vi "get property.vi"(0 "reference in":refnum<class "TDMS_DataHandler.lvclass">, 2 "Combo Box":T1, 5 "error in (no error)":errorcluster) -> (14 "reference out":refnum<class "TDMS_DataHandler.lvclass">, 16 "data":string, 19 "error out":errorcluster)   [LabVIEW 2019, in "TDMS_DataHandler.lvclass"]
uses:
  TDMS_DataHandler.lvclass
  PSnex TDMS fcurve property names.ctl
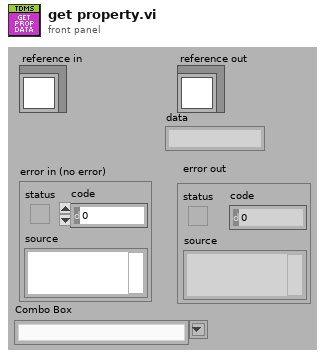
[diagram p1: front panel]
types:
  T1 = typedef "TDMS_DataHandler.lvclass/PSnex TDMS fcurve property names.ctl" = string
  T2 = typedef "TDMS_DataHandler.lvclass/ObjectAttributes.ctl" = cluster{"Directory":path, "FilePath":path, "FileRef":refnum<k34>, "ExperimentName":string, "GroupName":string, "ChannelNames":string[], "Datum":waveform(dbl)[], "Group_Metadata":cluster{"property names":string[], "property values":variant[]}, "Channel_Metadata":cluster{"property names":string[], "property values":variant[]}}
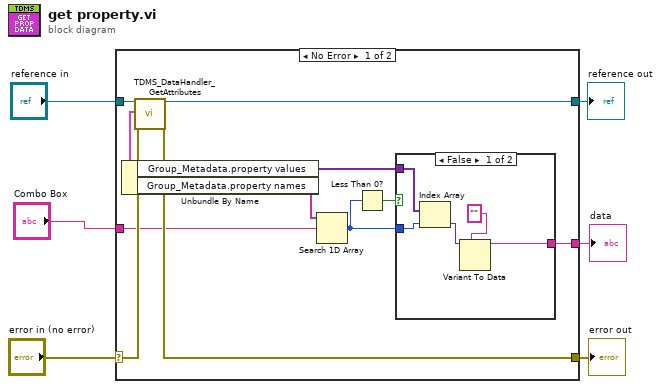
[diagram p0: block diagram]
diagram:
  n1 = case shown="No Error" "error in (no error)" {
    selector: "error in (no error)" -> [w17 w24]
    tunnel: [w16 w24] -> w5
    tunnel: [w15 w23] -> w3
    tunnel: "reference in" -> [w13 w23]
    tunnel: "Combo Box" -> [w11 _]
    tunnel: [w7 _] -> w1
    frame No Error {
      n2 = call "TDMS_DataHandler_GetAttributes.vi"("reference in"=w13, "error in (no error)"=w17) -> ("reference out"=w15:refnum<class "TDMS_DataHandler.lvclass">, "attributes"=w14:T2, "error out"=w16:errorcluster)  [unwired: 14 in, 1 out]
      n3 = Unbundle By Name(w14) -> ("Group_Metadata.property values"=w10:variant[], "Group_Metadata.property names"=w12:string[])
      n4 = Search 1D Array(1D array=w12, element=w11) -> (index of element=w9:i32)  [unwired: 1 in]
      n5 = Less Than 0?(x=w9) -> (x < 0?=w8:bool)
      n6 = case shown="False" w8 {
        tunnel: w10 -> [w22 _]
        tunnel: w9 -> [w21 _]
        tunnel: [w18 _] -> w7
        frame False {
          n7 = Index Array(array=w22, index=w21) -> (element=w20:variant)
          n8 = Variant To Data(type="", Variant=w20) -> (data=w18:string)  [unwired: 1 in, 1 out]
        }
        frame True {
        }
      }
    }
    frame Error {
    }
  }
  "error out" <- w5
  "reference out" <- w3
  "data" <- w1
